vi "Arith4.vi"(9 "Operation":enum16{"Add", "Sub", "Mult", "Div"}(ring), 10 "B":dbl, 11 "A":dbl) -> (3 "Output":dbl)   [LabVIEW 2025]
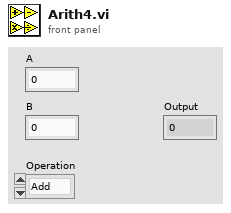
[diagram p1: front panel]
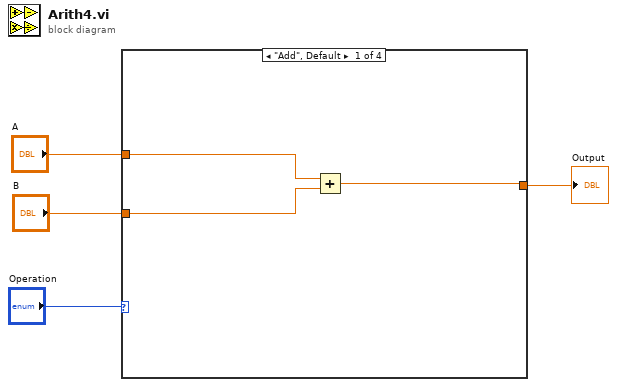
[diagram p0: block diagram]
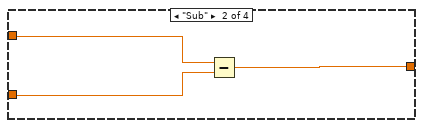
[diagram p2: hidden frame]
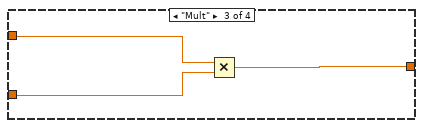
[diagram p3: hidden frame]
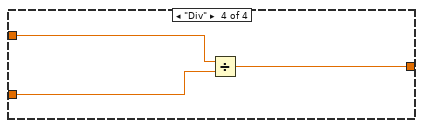
[diagram p4: hidden frame]
diagram:
  n1 = case shown="\"Add\", Default" "Operation" {
    tunnel: "A" -> [w7 w10 w12 w15]
    tunnel: "B" -> [w6 w9 w11 w14]
    tunnel: [w5 w8 w13 w16] -> w4
    frame "Add", Default {
      n2 = Add(x=w7, y=w6) -> (x+y=w5:dbl)
    }
    frame "Sub" {
      n3 = Subtract(x=w10, y=w9) -> (x-y=w8:dbl)
    }
    frame "Mult" {
      n4 = Multiply(x=w12, y=w11) -> (x*y=w13:dbl)
    }
    frame "Div" {
      n5 = Divide(x=w15, y=w14) -> (x/y=w16:dbl)
    }
  }
  "Output" <- w4
